vi "ExpressBlocks.vi"() -> ()   [LabVIEW 2015]
panel:
  out "Sine":dynamicdata(graph)
  out "RMS":dbl
  out "Positive Peak":dbl
  out "Negative Peak":dbl
  in  "Amplitude":dbl=1.0
  in  "Frequency":dbl=10.1
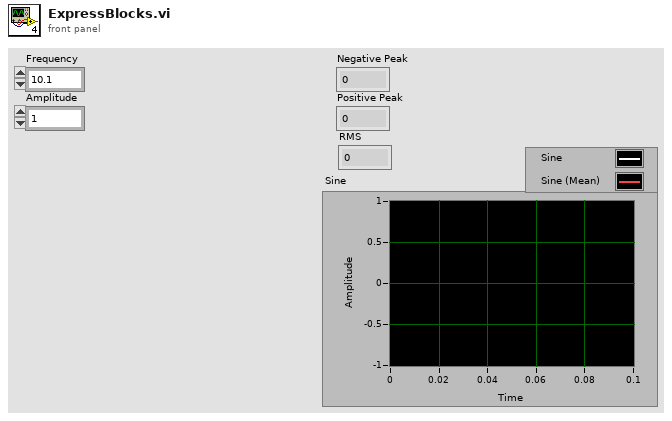
[diagram p1: front panel]
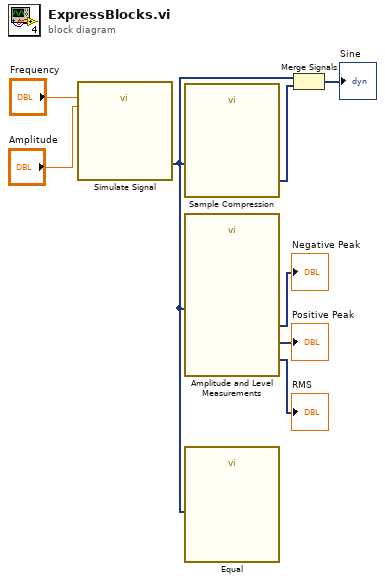
[diagram p0: block diagram]
diagram:
  n1 = call "Simulate Signal"("Frequency"="Frequency", "Amplitude"="Amplitude") -> ("Sine"=w1:dynamicdata)  [unwired: 12 in, 1 out]
  n2 = call "Sample Compression"("Signals"=w1) -> ("Mean"=w2:dynamicdata)  [unwired: 8 in, 2 out]
  n3 = call "Amplitude and Level Measurements"("Signals"=w1) -> ("RMS"=→"RMS":dynamicdata, "Negative Peak"=→"Negative Peak":dynamicdata, "Positive Peak"=→"Positive Peak":dynamicdata)  [unwired: 11 in, 1 out]
  n4 = call "Equal"("Operand 1"=w1) -> ()  [unwired: 9 in, 2 out]
  n5 = Merge Signals(w1, w2) -> (→"Sine":dynamicdata)
